vi "Test Validate HS256.vi"() -> ()   [LabVIEW 2015]
uses:
  JWT/JWT/JWT.lvclass
  JWT/Signature Algorithms.ctl
  JWT/JWT.lvlib
  JWT/Algorithm Key Pairs.ctl
panel:
  out "error out":errorcluster
  out "Valid?":bool
  in  "Key":string="blah"
  in  "Token":string="eyJhbGciOiJIUzI1NiIsInR5cCI6IkpXVCJ9.eyJzdWIiOiIxMjM0NTY3ODkwIiwibmFtZSI6IkpvaG4gRG9lIiwiaWF0IjoxNTE2MjM5MDIyfQ.gKf4Roky3w9YGQCP5qSwYkuksuijhL5M5ySONP0h5Z8"
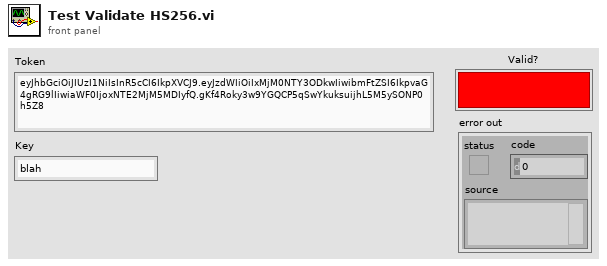
[diagram p1: front panel]
types:
  T1 = typedef "JWT.lvlib/Signature Algorithms.ctl" = enum16{"none", "HS256"}
  T2 = typedef "JWT.lvlib/Algorithm Key Pairs.ctl" = cluster{"Algs":T1[], "Keys":string[]}
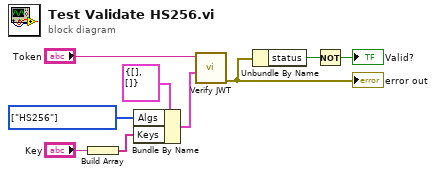
[diagram p0: block diagram]
diagram:
  w7 = T1[] [enum."HS256"] items=["none", "HS256"] ("Algs")
  n1 = Build Array("Key") -> (w5:string[])
  n2 = Bundle By Name(cluster=T2 {"Algs"=[], "Keys"=[]} ("Algorithm Key Pair"), "Algs"=w7, "Keys"=w5) -> (w4:T2)
  n3 = call "Verify JWT.vi"("Approved Algs"=w4, "Token"="Token") -> ("error out"=w3:errorcluster)  [unwired: 8 in, 1 out]
  "error out" <- w3
  n4 = Unbundle By Name(w3) -> ("status"=w2:bool)
  n5 = Not(x=w2) -> (.not. x?=→"Valid?":bool)
